vi "TestOPC.vi"   [LabVIEW 2014]
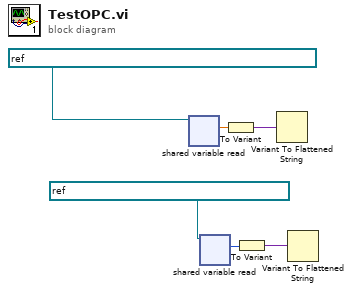
[diagram p0: block diagram]
diagram:
  n1 = shared-variable-read(refnum<k21> "ni.var.psp://My Computer/TestOPC/192.168.3.39_test" ("shared variable refnum in")) -> (w4:dbl)  [unwired: 1 in, 2 out]
  n2 = shared-variable-read(refnum<k21> "ni.var.psp://My Computer/TestOPC/test" ("shared variable refnum in")) -> (w3:u16)  [unwired: 1 in, 2 out]
  n3 = To Variant(anything=w4) -> (Variant=w2:variant)
  n4 = To Variant(anything=w3) -> (Variant=w1:variant)
  n5 = Variant To Flattened String(Variant=w2) -> ()  [unwired: 2 out]
  n6 = Variant To Flattened String(Variant=w1) -> ()  [unwired: 2 out]
